vi "fetch_samples.vi"(8 "error in (no error)":errorcluster, 11 "GenericToplevelComponent in":refnum<class "GenericToplevelComponent.lvclass">) -> (0 "error out":errorcluster, 2 "channels raw data block":T1, 3 "GenericToplevelComponent out":refnum<class "GenericToplevelComponent.lvclass">, 4 "# elements in queue":i32)   [LabVIEW 2010, in "GenericToplevelComponent.lvclass"]
uses:
  GenericToplevelComponent.lvclass
  arrays/pixel_raw_data_array.ctl
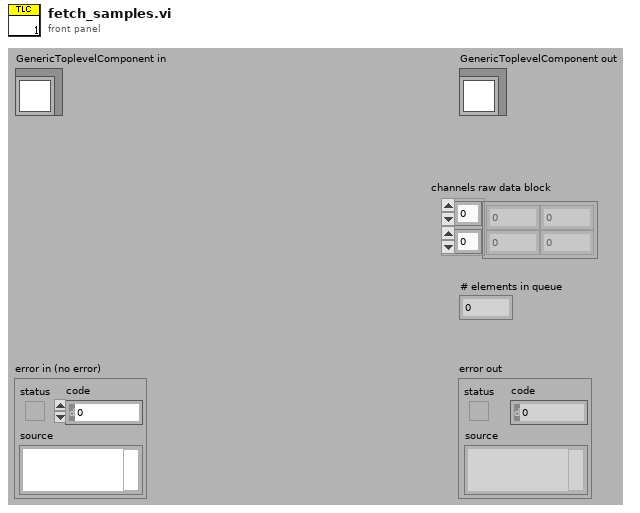
[diagram p1: front panel]
types:
  T1 = typedef "pixel_raw_data_array.ctl" = dbl[][]
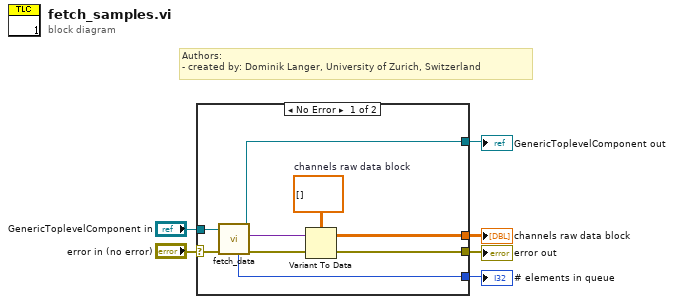
[diagram p0: block diagram]
diagram:
  # "Authors: \n- created by: Dominik Langer, University of Zurich, Switzerland"
  n1 = case shown="No Error" "error in (no error)" {
    selector: "error in (no error)" -> [w14 w17]
    tunnel: [w13 w17] -> w5
    tunnel: [w9 w16] -> w3
    tunnel: "GenericToplevelComponent in" -> [w10 w16]
    tunnel: [w8 _] -> w2
    tunnel: [w7 _] -> w1
    frame No Error {
      w11 = T1 []  # channels raw data block
      n2 = call-dynamic "fetch_data.vi"("error in (no error)"=w14, "GenericToplevelComponent in"=w10) -> ("error out"=w15:errorcluster, "data out"=w12:variant, "GenericToplevelComponent out"=w9:refnum<class "GenericToplevelComponent.lvclass">, "# elements in queue"=w8:i32)  [unwired: 6 in]
      n3 = Variant To Data(error in=w15, Variant=w12, type=w11) -> (error out=w13:errorcluster, data=w7:T1)
    }
    frame Error {
    }
  }
  "error out" <- w5
  "GenericToplevelComponent out" <- w3
  "channels raw data block" <- w1
  "# elements in queue" <- w2
